vi "CAN Flatten.vi"(7 "payload in":u8[](array[numeric]), 8 "error in (no error)":errorcluster, 10 "Data in":T1[](array[typedef]) {"Tags" format="%.0x"; "payload" format="%x"; "identifier" format="%x"}, 11 "CIFFifo in":refnum<class "CIFfifo.lvclass">) -> (0 "error out":errorcluster, 2 "Data out":T1[](array[typedef]) {"Tags" format="%.0x"; "payload" format="%x"; "identifier" format="%x"}, 3 "CIFFifo out":refnum<class "CIFfifo.lvclass">, 5 "payload out":u8[](array[numeric]))   [LabVIEW 2021, in "CIFfifo.lvclass"]
uses:
  CIFfifo.lvclass
  typedef/Datatype CAN.ctl
  CIFfifo.lvclass/CIFfifo.ctl
  be899675-9489-4ae7-9bdb-bbc908cd9623.vi
  fa4e04b0-1c28-4039-87e0-9391600efeb5.vi
  24dfac9c-4f7b-471b-adb6-3e40fb284e05.vi
  Accessors/Write Payload Length.vi
  Accessors/Read Header.vi
  CIFCore/Common/Utilities/Add Error.vi
  be899675-9489-4ae7-9bdb-bbc908cd9623.vi/c28b0ead-42ad-4072-80a2-aca7f2bd7ce3.vi
  fa4e04b0-1c28-4039-87e0-9391600efeb5.vi/c28b0ead-42ad-4072-80a2-aca7f2bd7ce3.vi
  24dfac9c-4f7b-471b-adb6-3e40fb284e05.vi/c28b0ead-42ad-4072-80a2-aca7f2bd7ce3.vi
  CIFCore/Common/Utilities/Append Error Location.vi
  ChannelCommon.lvlib
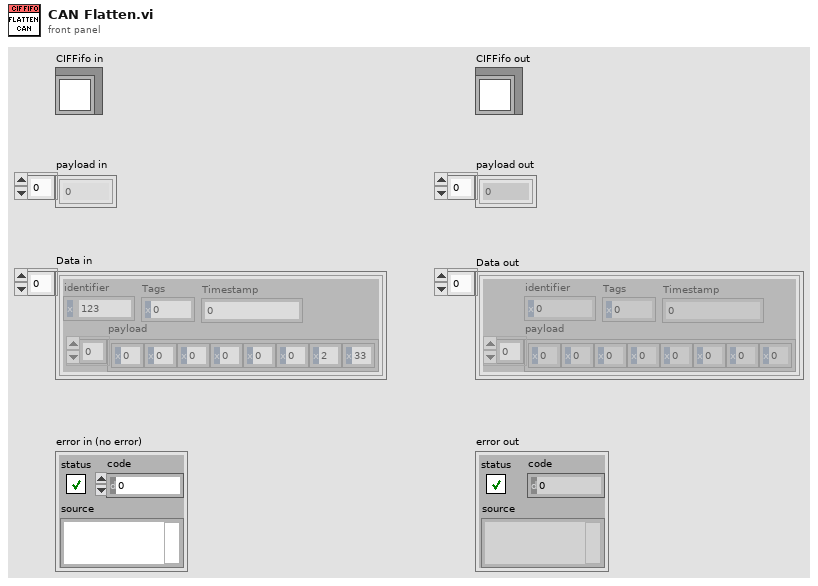
[diagram p1: front panel]
types:
  T1 = typedef "ChannelCommon.lvlib/Datatype CAN.ctl" = cluster{"payload":u8[], "identifier":u32, "Tags":u8, "Timestamp":u64}
  T2 = typedef "ChannelCommon.lvlib/FIFO Header.ctl" = cluster{"Length":u64, "T0":u64, "T_Out":u64, "T_Tx":u64, "Ctr":u64, "ClockID":u8}
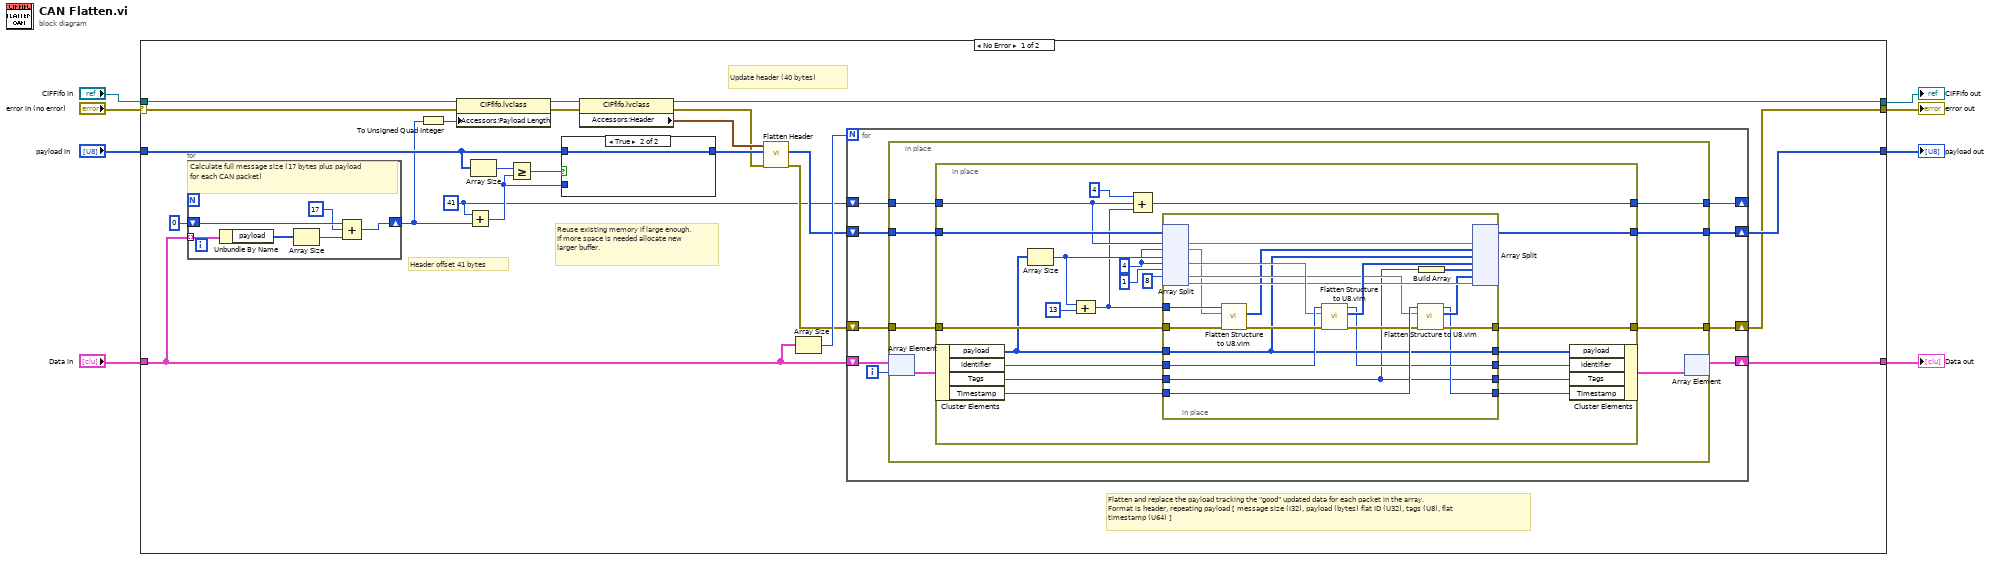
[diagram p0: block diagram]
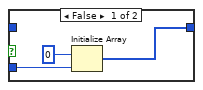
[diagram p2: hidden frame]
diagram:
  n1 = case shown="No Error" "error in (no error)" {
    selector: "error in (no error)" -> [w21 w103]
    tunnel: [w11 w103] -> w7
    tunnel: "Data in" -> [w14 w102]
    tunnel: [w10 w102] -> w5
    tunnel: "CIFFifo in" -> [w30 w101]
    tunnel: [w13 w101] -> w1
    tunnel: [w12 w100] -> w3
    tunnel: "payload in" -> [w22 w100]
    frame No Error {
      w9 = 41 ("y")
      # "Flatten and replace the payload tracking the \"good\" updated data for each packet in the array.\nFormat is header, repeating payload [ message size (I32), payload (bytes) flat ID (U32), tags (U8), flat timestamp (U64) ]"
      # "Header offset 41 bytes"
      # "Update header (40 bytes)"
      # "Reuse existing memory if large enough.  If more space is needed allocate new larger buffer."
      n2 = for {
        tunnel: w14 -> [w99] mode=indexing
        shift-right: [w97] -> w20
        shift-left: 0 -> [w96]
        # "Calculate full message size (17 bytes plus payload for each CAN packet)"
        n3 = Unbundle By Name(w99) -> ("payload"=w98:u8[])
        n4 = Array Size(array=w98) -> (size(s)=w95:i32)
        n5 = Compound Arithmetic op=ADD(w96, 17 ("value"), w95) -> (w97:i32)
      }
      n6 = To Unsigned Quad Integer(1:w20) -> (0:w28:u64)
      n7 = property class="CIFfifo.lvclass"(reference=w30, error in=w21, "Accessors:Payload Length"=w28) -> (reference out=w19:refnum<class "CIFfifo.lvclass">, error out=w18:errorcluster)
      n8 = Add(x=w9, y=w20) -> (x+y=w23:i32)
      n9 = Array Size(array=w22) -> (size(s)=w27:i32)
      n10 = Greater Or Equal?(x=w27, y=w23) -> (x >= y?=w26:bool)
      n11 = case shown="True" w26 {
        tunnel: w22 -> [_ w93]
        tunnel: [w90 w93] -> w25
        tunnel: w23 -> [w92 _]
        frame False {
          n12 = Initialize Array(u8 0, w92) -> (w90:u8[])
        }
        frame True {
        }
      }
      n13 = property class="CIFfifo.lvclass"(reference=w19, error in=w18) -> (reference out=w13:refnum<class "CIFfifo.lvclass">, error out=w24:errorcluster, "Accessors:Header"=w29:T2)
      n14 = call "Flatten Header.vi"("error in"=w24, "Flattened Data in"=w25, "Header in"=w29) -> ("error out"=w15:errorcluster, "Flattened Data out"=w16:u8[])  [unwired: 6 in, 1 out]
      n15 = Array Size(array=w14) -> (size(s)=w17:i32)
      n16 = for {
        N: w17 -> [_]
        shift-right: [w40] -> w11
        shift-left: w15 -> [w39]
        shift-right: [w37] -> w12
        shift-left: w16 -> [w38]
        shift-right: [w35] -> _
        shift-left: w9 -> [w36]
        shift-right: [w32] -> w10
        shift-left: w14 -> [w34]
        i -> [w33]
        n17 = in-place {
          in-place-border: [w48] -> w40
          in-place-border: w39 -> [w47]
          in-place-border: w38 -> [w46]
          in-place-border: [w45] -> w37
          in-place-border: w36 -> [w44]
          in-place-border: [w43] -> w35
          n18 = in-place-array #1(w34, w33) -> (w42:T1)
          n19 = in-place {
            in-place-border: [w69] -> w48
            in-place-border: w47 -> [w68]
            in-place-border: w46 -> [w67]
            in-place-border: [w66] -> w45
            in-place-border: w44 -> [w65]
            in-place-border: [w64] -> w43
            w59 = 4
            n20 = in-place-cluster #2(w42) -> ("payload"=w56:u8[], "identifier"=w55:u32, "Tags"=w50:u8, "Timestamp"=w54:u64)
            n21 = Array Size(array=w56) -> (size(s)=w60:i32)
            n22 = Compound Arithmetic op=ADD(w60, 13 ("value")) -> (w58:i32)
            n23 = Compound Arithmetic op=ADD(4, w65, w58) -> (w64:i32)
            n24 = in-place {
              in-place-border: w54 -> [w86]
              in-place-border: w68 -> [w88]
              in-place-border: [w87] -> w69
              in-place-border: w56 -> [w74]
              in-place-border: w55 -> [w83]
              in-place-border: w58 -> [w77]
              in-place-border: [w74] -> w53
              in-place-border: [w73] -> w52
              in-place-border: [w72] -> w51
              in-place-border: w50 -> [w70]
              in-place-border: [w70] -> w49
              n25 = in-place-split #3(w67, w65, w59, w60, w59, 1, 8) -> (w89:u8[], w75:u8[], w82:u8[], w79:u8[], w80:u8[])  [unwired: 2 out]
              n26 = call "Flatten Structure to U8.vim"("error in"=w88, "Flattened Data in"=w75, "Data to Flatten in"=w77) -> ("error out"=w85:errorcluster, "Flattened Data out"=w76:u8[])  [unwired: 6 in, 1 out]
              n27 = call "Flatten Structure to U8.vim"("error in"=w85, "Flattened Data in"=w82, "Data to Flatten in"=w83) -> ("error out"=w84:errorcluster, "Flattened Data out"=w81:u8[], "Data to Flatten out"=w73:u32)  [unwired: 6 in]
              n28 = call "Flatten Structure to U8.vim"("error in"=w84, "Flattened Data in"=w79, "Data to Flatten in"=w86) -> ("error out"=w87:errorcluster, "Flattened Data out"=w78:u8[], "Data to Flatten out"=w72:u64)  [unwired: 6 in]
              n29 = Build Array(w70) -> (w71:u8[])
              n30 = in-place-split #3(w89, w76, w74, w81, w71, w78, w80) -> (w66:u8[])  [unwired: 6 out]
            }
            n31 = in-place-cluster #2("payload"=w53, "identifier"=w52, "Tags"=w49, "Timestamp"=w51) -> (w41:T1)
          }
          n32 = in-place-array #1(w41) -> (w32:T1[])  [unwired: 1 out]
        }
      }
    }
    frame Error {
    }
  }
  "error out" <- w7
  "Data out" <- w5
  "CIFFifo out" <- w1
  "payload out" <- w3
